vi "Write shift.vi"(10 "shift":i64, 11 "Node in":refnum<class "Node.lvclass">) -> (3 "Node out":refnum<class "Node.lvclass">)   [LabVIEW 2023, in "d20.lvlib" / "Node.lvclass"]
uses:
  Node.lvclass
  Node.lvclass/Node.ctl
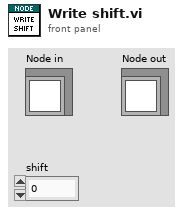
[diagram p1: front panel]
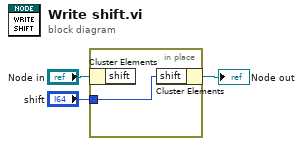
[diagram p0: block diagram]
diagram:
  n1 = in-place {
    in-place-border: "shift" -> [w4]
    n2 = in-place-cluster #1("Node in") -> ()  [unwired: 1 out]
    n3 = in-place-cluster #1("shift"=w4) -> (→"Node out":refnum<class "Node.lvclass">)
  }
